vi "StringArray Destroy.vi"(8 "error in (no error)":errorcluster, 11 "StringArray DVR in":refnum<data-value>) -> (0 "error out":errorcluster)   [LabVIEW 2012, in "MDSplus.lvlib"]
uses:
  <vilib>/MDSplus/Library/MDSplus.lvlib
  <vilib>/MDSplus/Classes/Data_Class/Array_Class/StringArray_Class/StringArray.lvclass
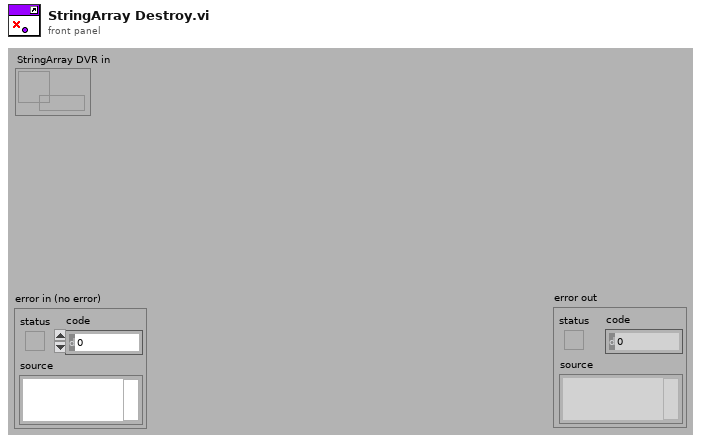
[diagram p1: front panel]
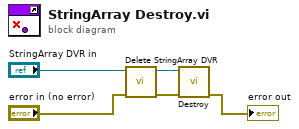
[diagram p0: block diagram]
diagram:
  n1 = call <vilib>:"Delete StringArray DVR.vi"("error in (no error)"="error in (no error)", "StringArray DVR in"="StringArray DVR in") -> ("error out"=w2:errorcluster, "StringArray out"=w3:refnum<class "StringArray.lvclass">)  [unwired: 8 in]
  n2 = call-dynamic "Destroy.vi"("error in (no error)"=w2, "StringArray in"=w3) -> ("error out"=→"error out":errorcluster)  [unwired: 9 in]
